vi "Insert FileName In Error.vi"(3 "error in":errorcluster, 4 "Path":path) -> (5 "error out":errorcluster)   [LabVIEW 2025, in "XNode Support.lvlib"]
uses:
  XNode Support.lvlib
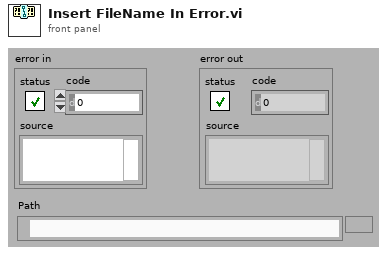
[diagram p1: front panel]
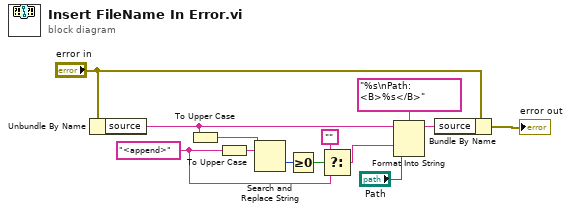
[diagram p0: block diagram]
diagram:
  w4 = "<append>" ("search string")
  n1 = Unbundle By Name("error in") -> ("source"=w13:string)
  n2 = To Upper Case(1:w13) -> (0:w1:string)
  n3 = To Upper Case(1:w4) -> (0:w2:string)
  n4 = Search and Replace String(input string=w1, search string=w2) -> (offset past replacement=w6:i32)  [unwired: 6 in, 3 out]
  n5 = Greater Or Equal To 0?(x=w6) -> (x >= 0?=w7:bool)
  n6 = Select(t="", s=w7, f=w4) -> (s? t:f=w3:string)
  n7 = Format Into String(format string="%s\nPath: <B>%s</B>", initial string=w13, w3, "Path") -> (resulting string=w8:string)  [unwired: 1 in, 1 out]
  n8 = Bundle By Name(cluster="error in", "source"=w8) -> (→"error out":errorcluster)
